vi "测量流程.vi"(11 "控制命令":T1(ring)) -> ()   [LabVIEW 2016, in "斯坦道总磷总氮.lvlib"]
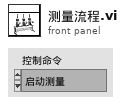
[diagram p1: front panel]
types:
  T1 = enum16{"启动测量", "标样核查", "零点核查", "跨度核查", "空白测试", "平行样测试", "加标回收", "空白校准", "标样校准", "初始化（清洗）", "停止测试", "仪器重启", "校时", "模式设置", "测量间隔设置"}
  T2 = cluster{"COD":bool, "氨氮":bool, "总氮":bool, "总磷":bool}
  T3 = cluster{"站号":u16, "量程切换":enum32{"H", "L", "AUTO"}, "控制命令":enum16{"启动测量", "标样核查", "零点核查", "跨度核查", "空白测试", "平行样测试", "加标回收", "空白校准", "标样校准", "初始化（清洗）", "停止测试", "仪器重启", "校时", "模式设置", "测量间隔设置"}, "模式设置":enum16{"待机", "连续模式", "周期模式", "定点模式", "受控模式", "手动模式"}, "测量间隔":u16}
  T4 = cluster{"时间标识":timestamp, "设备":string, "日志信息":string, "流程参数":string}
  T5 = enum16{"空闲", "水样测试", "标样核查", "零点核查", "跨度核查", "空白测试", "平行样测试", "加标回收", "空白校准", "标样校准", "初始化（清洗）"}
  T6 = cluster{"系统时间":timestamp, "工作状态":enum16{"空闲", "水样测试", "标样核查", "零点核查", "跨度核查", "空白测试", "平行样测试", "加标回收", "空白校准", "标样校准", "初始化（清洗）"}, "测量模式":enum16{"待机", "连续模式", "周期模式", "定点模式", "受控模式", "手动模式"}, "告警代码":u16, "故障代码":u16, "日志代码":u16, "软件版本":u16, "F0":sgl, "F1":sgl, "F2":sgl, "F3":sgl, "T":sgl, "H":sgl, "id":u16, "flowid":u16, "量程":u16, "总磷控温温度1":sgl, "营养盐控温温度2":sgl, "ADC":sgl}
  T7 = cluster{"水样测试量程模式":enum16{"H", "L", "AUTO"}, "空白核查量程模式":enum16{"H", "L", "AUTO"}, "跨度核查量程模式":enum16{"H", "L", "AUTO"}, "加标回收量程模式":enum16{"H", "L", "AUTO"}}
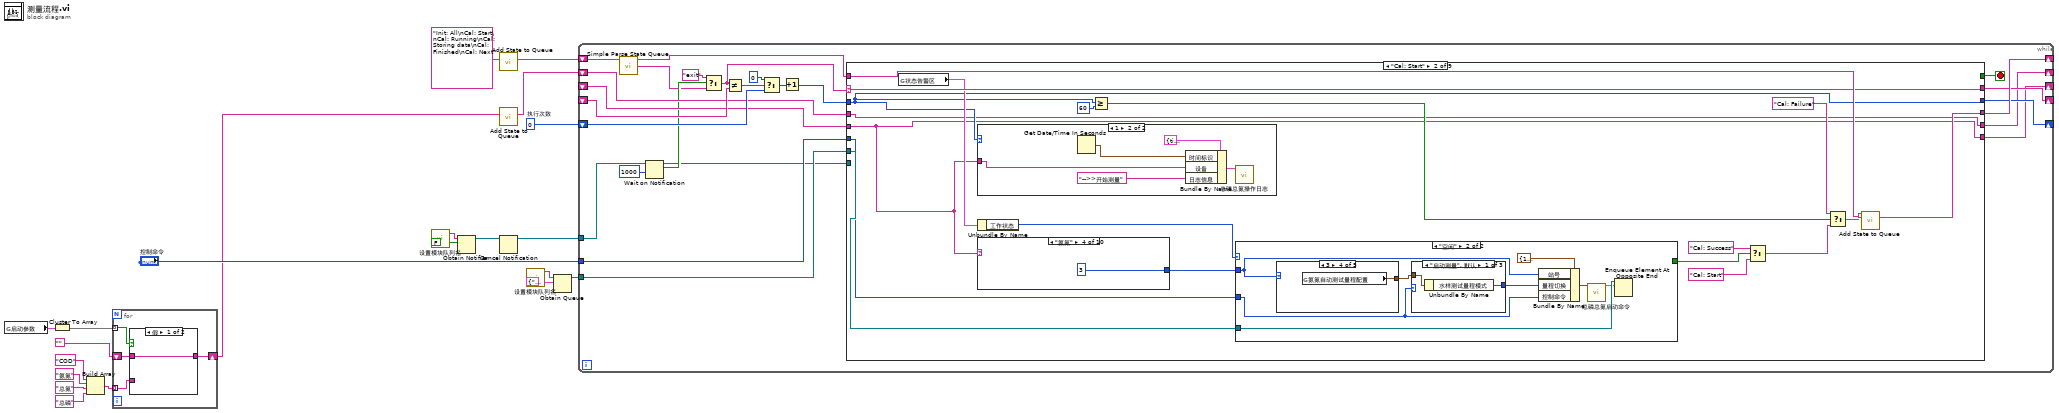
[diagram p0: block diagram]
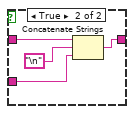
[diagram p2: hidden frame]
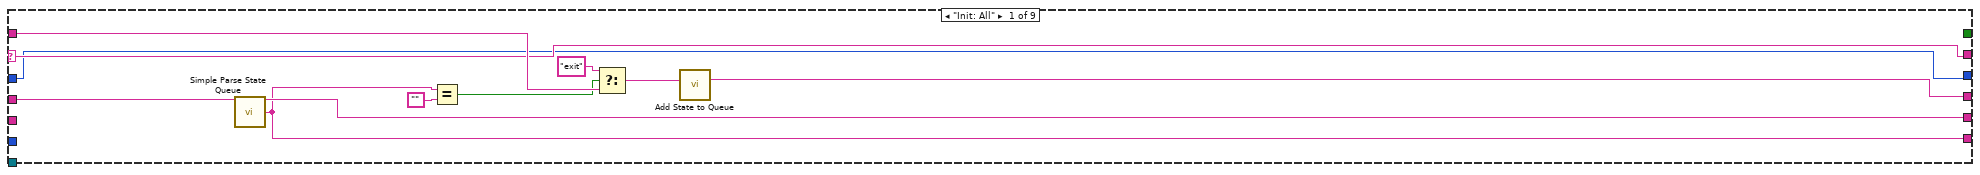
[diagram p3: hidden frame]
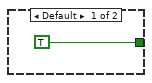
[diagram p4: hidden frame]
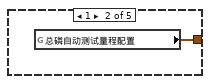
[diagram p6: hidden frame]
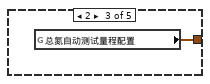
[diagram p7: hidden frame]
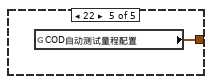
[diagram p8: hidden frame]
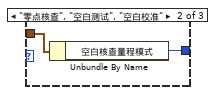
[diagram p9: hidden frame]
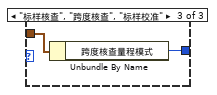
[diagram p10: hidden frame]
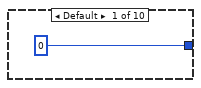
[diagram p11: hidden frame]
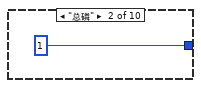
[diagram p12: hidden frame]
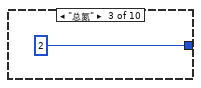
[diagram p13: hidden frame]
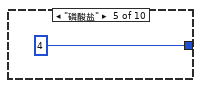
[diagram p14: hidden frame]
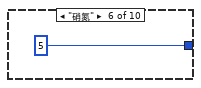
[diagram p15: hidden frame]
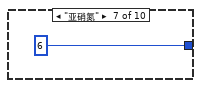
[diagram p16: hidden frame]
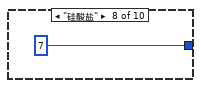
[diagram p17: hidden frame]
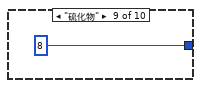
[diagram p18: hidden frame]
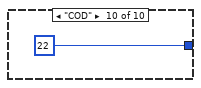
[diagram p19: hidden frame]
diagram:
  w15 = 0  # 执行次数
  n1 = global read "总磷总氮断电保存全局变量.vi" "启动参数"() -> (w9:T2)
  n2 = Cluster To Array(cluster=w9) -> (array=w1:bool[])
  n3 = Build Array("COD", "氨氮", "总氮", "总磷") -> (w6:string[])
  n4 = for {
    tunnel: w1 -> [w22] mode=indexing
    tunnel: w6 -> [w23] mode=indexing
    shift-right: [w24] -> w4
    shift-left: "" -> [w25]
    n5 = case shown="假" w22 {
      tunnel: w25 -> [w26 w30]
      tunnel: [w26 w29] -> w24
      tunnel: w23 -> [_ w28]
      frame False {
      }
      frame True {
        n6 = Concatenate Strings(w30, "\n", w28) -> (w29:string)
      }
    }
  }
  n7 = call "设置模块队列名.vi"() -> ("Msg"=w12:string)  [unwired: 5 in]
  n8 = Obtain Notifier(name (unnamed)=w12, notification data type=FALSE) -> (notifier out=w20:refnum<notifier>)  [unwired: 2 in, 2 out]
  n9 = call "Add State to Queue.vi"("State(s) In (\"\")"="Init: All\nCal: Start\nCal: Running\nCal: Storing data\nCal: Finished\nCal: Next" ("State(s) In (\"\")")) -> ("States Out"=w18:string)  [unwired: 14 in]
  n10 = call "Add State to Queue.vi"("State(s) In (\"\")"=w4) -> ("States Out"=w13:string)  [unwired: 14 in]
  n11 = Cancel Notification(0:w20) -> (8:w10:refnum<notifier>)  [unwired: 1 in, 2 out]
  n12 = call "设置模块队列名.vi"() -> ("Msg"=w11:string)  [unwired: 5 in]
  n13 = Obtain Queue(name (unnamed)=w11, element data type=cluster{"命令":string, "data":variant} {"命令"="", "data"=variant}) -> (queue out=w16:refnum<queue>)  [unwired: 3 in, 2 out]
  n14 = while {
    tunnel: w16 -> [w53]
    shift-right: [w52] -> _
    shift-left: w18 -> [w55]
    shift-right: [w45] -> _
    shift-left: w15 -> [w48]
    shift-right: [w51] -> _
    shift-left: _ -> [w50]
    tunnel: "控制命令" -> [w43]
    shift-right: [w39] -> _
    shift-left: w13 -> [w41]
    shift-right: [w40] -> _
    shift-left: _ -> [w38]
    tunnel: w10 -> [w36]
    stop <- w42 stop-if-true
    n15 = call "Simple Parse State Queue.vi"("State Queue"=w55) -> ("Remain States"=w54:string, "Next State"=w33:string)  [unwired: 13 in]
    n16 = Wait on Notification(notifier=w36, timeout in ms (-1)=1000 ("超时毫秒(-1)")) -> (notifier out=w31:refnum<notifier>, notification=w35:bool)  [unwired: 2 in, 2 out]
    n17 = Select(t="exit", s=w35, f=w33) -> (s? t:f=w32:string)
    n18 = Not Equal?(x=w32, y=w50) -> (x != y?=w49:bool)
    n19 = Select(t=0, s=w49, f=w48) -> (s? t:f=w46:i32)
    n20 = Increment(x=w46) -> (x+1=w44:i32)
    n21 = case shown="\"Cal: Start\"" w32 {
      selector: w32 -> [w62 w83 w123 w138 w144 w158 w174 w185 w192]
      tunnel: w54 -> [w64 w85 w125 _ w155 w163 w176 _ w193]
      tunnel: w53 -> [_ w81 _ _ _ _ _ _ w188]
      tunnel: [w66 w84 w124 w139 w154 w162 w175 "Init: All\nCal: Start\nCal: Running\nCal: Storing data\nCal: Finished\nCal: Next" ("State(s) In (\"\")") w193] -> w52
      tunnel: [w62 w83 w123 w138 w144 w158 w174 w185 w192] -> w51
      tunnel: [w61 w78 w122 w137 w147 w161 w172 w184 w191] -> w45
      tunnel: w44 -> [w61 w78 w122 w137 w147 w161 w172 w184 w191]
      tunnel: w43 -> [_ w80 _ _ _ _ _ _ _]
      tunnel: [_ _ _ _ _ _ _ _ TRUE] -> w42
      tunnel: w41 -> [w60 w67 w121 w131 w141 w165 w173 w183 w190]
      tunnel: [w58 w68 w120 w130 w140 w164 w171 w182 w189] -> w40
      tunnel: [w59 w67 w121 w131 w141 w165 w173 w183 w190] -> w39
      tunnel: w38 -> [_ w68 w120 w130 w140 w164 w171 w182 w189]
      tunnel: w31 -> [_ _ _ _ _ _ _ _ w187]
      frame "Init: All" {
        n22 = call "Simple Parse State Queue.vi"("State Queue"=w60) -> ("Remain States"=w59:string, "Next State"=w58:string)  [unwired: 13 in]
        n23 = Equal?(x=w58, y="") -> (x = y?=w56:bool)
        n24 = Select(t="exit", s=w56, f=w64) -> (s? t:f=w63:string)
        n25 = call "Add State to Queue.vi"("State(s) In (\"\")"=w63) -> ("States Out"=w66:string)  [unwired: 14 in]
      }
      frame "Cal: Start" {
        n26 = global read "VAR总磷总氮全局变量.vi" "状态告警区"() -> (w82:T6)
        n27 = case shown="1" w78 {
          tunnel: w68 -> [_ w115]
          frame 0, Default {
          }
          frame 1 {
            n28 = Get Date/Time In Seconds() -> (seconds since 1Jan1904=w119:timestamp)
            n29 = Bundle By Name(cluster=T4 {"时间标识"=timestamp(0 s since 1904-01-01), "设备"="", "日志信息"="", "流程参数"=""} ("data in"), "时间标识"=w119, "设备"=w115, "日志信息"="-->>开始测量") -> (w118:T4)
            n30 = call "总磷总氮操作日志.vi"("data in"=w118) -> ()  [unwired: 11 in]
          }
        }
        n31 = Unbundle By Name(w82) -> ("工作状态"=w69:T5)
        n32 = case shown="\"氨氮\"" w68 {
          tunnel: [0 1 2 3 4 5 6 7 8 22] -> w79
          frame Default {
          }
          frame "总磷" {
          }
          frame "总氮" {
          }
          frame "氨氮" {
          }
          frame "磷酸盐" {
          }
          frame "硝氮" {
          }
          frame "亚硝氮" {
          }
          frame "硅酸盐" {
          }
          frame "硫化物" {
          }
          frame "COD" {
          }
        }
        n33 = Greater Or Equal?(x=w78, y=60) -> (x >= y?=w76:bool)
        n34 = case shown="\"空闲\"" w69 {
          tunnel: w80 -> [_ w90]
          tunnel: w81 -> [_ w93]
          tunnel: [TRUE _] -> w73
          tunnel: w79 -> [_ w88]
          frame Default {
          }
          frame "空闲" {
            n35 = case shown="3" w88 {
              tunnel: [_ w95 w96 w97 w98] -> w89
              frame 0, Default {
              }
              frame 1 {
                n36 = global read "总磷总氮断电保存全局变量.vi" "总磷自动测试量程配置"() -> (w95:T7)
              }
              frame 2 {
                n37 = global read "总磷总氮断电保存全局变量.vi" "总氮自动测试量程配置"() -> (w96:T7)
              }
              frame 3 {
                n38 = global read "总磷总氮断电保存全局变量.vi" "氨氮自动测试量程配置"() -> (w97:T7)
              }
              frame 22 {
                n39 = global read "总磷总氮断电保存全局变量.vi" "COD自动测试量程配置"() -> (w98:T7)
              }
            }
            n40 = case shown="\"启动测量\", 默认" w90 {
              tunnel: w89 -> [w100 w102 w104]
              tunnel: [w99 w101 w103] -> w94
              frame "启动测量", Default {
                n41 = Unbundle By Name(w100) -> ("水样测试量程模式"=w99:enum16{"H", "L", "AUTO"})
              }
              frame "零点核查", "空白测试", "空白校准" {
                n42 = Unbundle By Name(w102) -> ("空白核查量程模式"=w101:enum16{"H", "L", "AUTO"})
              }
              frame "标样核查", "跨度核查", "标样校准" {
                n43 = Unbundle By Name(w104) -> ("跨度核查量程模式"=w103:enum16{"H", "L", "AUTO"})
              }
            }
            n44 = Bundle By Name(cluster=T3 {"站号"=1, "量程切换"=enum."AUTO", "控制命令"=enum."启动测量", "模式设置"=enum."待机", "测量间隔"=0} ("参数"), "站号"=w88, "量程切换"=w94, "控制命令"=w90) -> (w91:T3)
            n45 = call "总磷总氮启动命令.vi"("参数"=w91) -> ("启动命令"=w87:cluster{"命令":string, "data":variant})  [unwired: 10 in]
            n46 = Enqueue Element At Opposite End(queue=w93, element=w87) -> ()  [unwired: 2 in, 3 out]
          }
        }
        n47 = Select(t="Cal: Success" ("State(s) In (\"\")"), s=w73, f="Cal: Start" ("State(s) In (\"\")")) -> (s? t:f=w71:string)
        n48 = Select(t="Cal: Failure" ("State(s) In (\"\")"), s=w76, f=w71) -> (s? t:f=w74:string)
        n49 = call "Add State to Queue.vi"("State(s) In Front (\"\")"=w74, "State(s) In (\"\")"=w85) -> ("States Out"=w84:string)  [unwired: 13 in]
      }
      frame "Cal: Success" {
        n50 = Get Date/Time In Seconds() -> (seconds since 1Jan1904=w128:timestamp)
        n51 = Bundle By Name(cluster=T4 {"时间标识"=timestamp(0 s since 1904-01-01), "设备"="", "日志信息"="", "流程参数"=""} ("data in"), "时间标识"=w128, "设备"=w120, "日志信息"="-->>启动成功") -> (w127:T4)
        n52 = call "总磷总氮操作日志.vi"("data in"=w127) -> ()  [unwired: 11 in]
        n53 = call "Add State to Queue.vi"("State(s) In (\"\")"=w125) -> ("States Out"=w124:string)  [unwired: 14 in]
      }
      frame "Cal: Failure" {
        n54 = Get Date/Time In Seconds() -> (seconds since 1Jan1904=w135:timestamp)
        n55 = Bundle By Name(cluster=T4 {"时间标识"=timestamp(0 s since 1904-01-01), "设备"="", "日志信息"="", "流程参数"=""} ("data in"), "时间标识"=w135, "设备"=w130, "日志信息"="-->>启动失败") -> (w134:T4)
        n56 = call "总磷总氮操作日志.vi"("data in"=w134) -> ()  [unwired: 11 in]
        n57 = call "Add State to Queue.vi"("State(s) In (\"\")"="exit" ("State(s) In (\"\")")) -> ("States Out"=w139:string)  [unwired: 14 in]
      }
      frame "Cal: Running" {
        n58 = global read "VAR总磷总氮全局变量.vi" "状态告警区"() -> (w151:T6)
        n59 = Unbundle By Name(w151) -> ("工作状态"=w152:T5)
        n60 = Less Or Equal?(x=w147, y=7200) -> (x <= y?=w145:bool)
        n61 = Select(t=w144, s=w145, f="exit") -> (s? t:f=w143:string)
        n62 = Equal?(x=w152, y=T5."空闲") -> (x = y?=w150:bool)
        n63 = Select(t="", s=w150, f=w143) -> (s? t:f=w148:string)
        n64 = call "Add State to Queue.vi"("State(s) In Front (\"\")"=w148, "State(s) In (\"\")"=w155) -> ("States Out"=w154:string)  [unwired: 13 in]
      }
      frame "Cal: Storing data" {
        n65 = case shown="1" w161 {
          tunnel: w164 -> [_ w166]
          frame 0, Default {
          }
          frame 1 {
            n66 = Get Date/Time In Seconds() -> (seconds since 1Jan1904=w170:timestamp)
            n67 = Bundle By Name(cluster=T4 {"时间标识"=timestamp(0 s since 1904-01-01), "设备"="", "日志信息"="", "流程参数"=""} ("data in"), "时间标识"=w170, "设备"=w166, "日志信息"="-->>存储数据") -> (w169:T4)
            n68 = call "总磷总氮操作日志.vi"("data in"=w169) -> ()  [unwired: 11 in]
          }
        }
        n69 = Less Or Equal?(x=w161, y=10) -> (x <= y?=w159:bool)
        n70 = Select(t=w158, s=w159, f="") -> (s? t:f=w156:string)
        n71 = call "Add State to Queue.vi"("State(s) In Front (\"\")"=w156, "State(s) In (\"\")"=w163) -> ("States Out"=w162:string)  [unwired: 13 in]
      }
      frame "Cal: Finished" {
        n72 = call "Add State to Queue.vi"("State(s) In (\"\")"=w176) -> ("States Out"=w175:string)  [unwired: 14 in]
        n73 = case shown="1" w172 {
          tunnel: w171 -> [_ w177]
          frame 0, Default {
          }
          frame 1 {
            n74 = Get Date/Time In Seconds() -> (seconds since 1Jan1904=w181:timestamp)
            n75 = Bundle By Name(cluster=T4 {"时间标识"=timestamp(0 s since 1904-01-01), "设备"="", "日志信息"="", "流程参数"=""} ("data in"), "时间标识"=w181, "设备"=w177, "日志信息"="-->>测量结束") -> (w180:T4)
            n76 = call "总磷总氮操作日志.vi"("data in"=w180) -> ()  [unwired: 11 in]
          }
        }
      }
      frame "Cal: Next" {
      }
      frame "exit", Default {
        n77 = Release Queue(queue=w188) -> ()  [unwired: 2 in, 3 out]
        n78 = Release Notifier(notifier=w187) -> ()  [unwired: 2 in, 3 out]
      }
    }
  }
